vi "数据主动和反控发送.vi"() -> ()   [LabVIEW 2016, in "数据传输系统.lvlib"]
uses:
  <vilib>/ptbypt/NI_PtbyPt.lvlib
panel:
  out "QN":string
  out "队列中元素数量":i32
  out "元素":cluster{"命令编码CN":string, "QN":string}[](array[cluster])
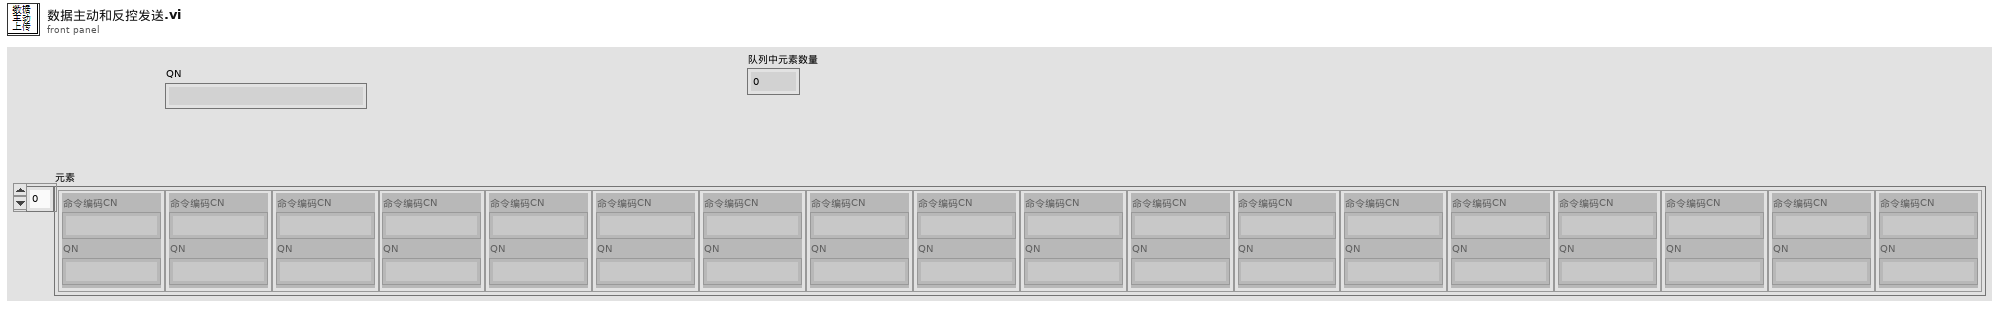
[diagram p1: front panel]
types:
  T1 = enum16{"00点", "01点", "02点", "03点", "04点", "05点", "06点", "07点", "08点", "09点", "10点", "11点", "12点", "13点", "14点", "15点", "16点", "17点", "18点", "19点", "20点", "21点", "22点", "23点"}
  T2 = enum16{"关闭", "星期日", "星期一", "星期二", "星期三", "星期四", "星期五", "星期六"}
  T3 = typedef "LVDateTimeRec.ctl" = cluster{"秒数的小数部分":dbl, "秒":i32, "分":i32, "时":i32, "日":i32, "月":i32, "年":i32, "天数（周）":i32, "天数（年）":i32, "DST":i32}
  T4 = cluster{"[0]":string, "[1]":string, "[2]":string, "[3]":string, "[4]":string, "[5]":string, "[6]":string, "[7]":string, "[8]":string, "[9]":string, "[10]":string, "[11]":string, "[12]":string, "[13]":string, "[14]":string, "[15]":string, "[16]":string, "[17]":string, "[18]":string, "[19]":string, "[20]":string, "[21]":string, "[22]":string, "[23]":string, "[24]":string, "[25]":string, "[26]":string}
  T5 = cluster{"CODMn":bool, "CODCr":bool, "DO":bool, "铜":bool, "PH":bool, "氨氮":bool, "比电导率":bool, "水温":bool, "COD":bool, "浊度":bool, "总氮":bool, "总磷":bool, "叶绿素a":bool, "藻密度":bool, "水位":bool, "流速":bool, "瞬时流量":bool, "累积流量":bool, "亚硝酸盐":bool, "硫化物":bool, "ORP":bool, "铅":bool, "镉":bool, "锌":bool, "镍":bool, "锰":bool, "汞":bool}
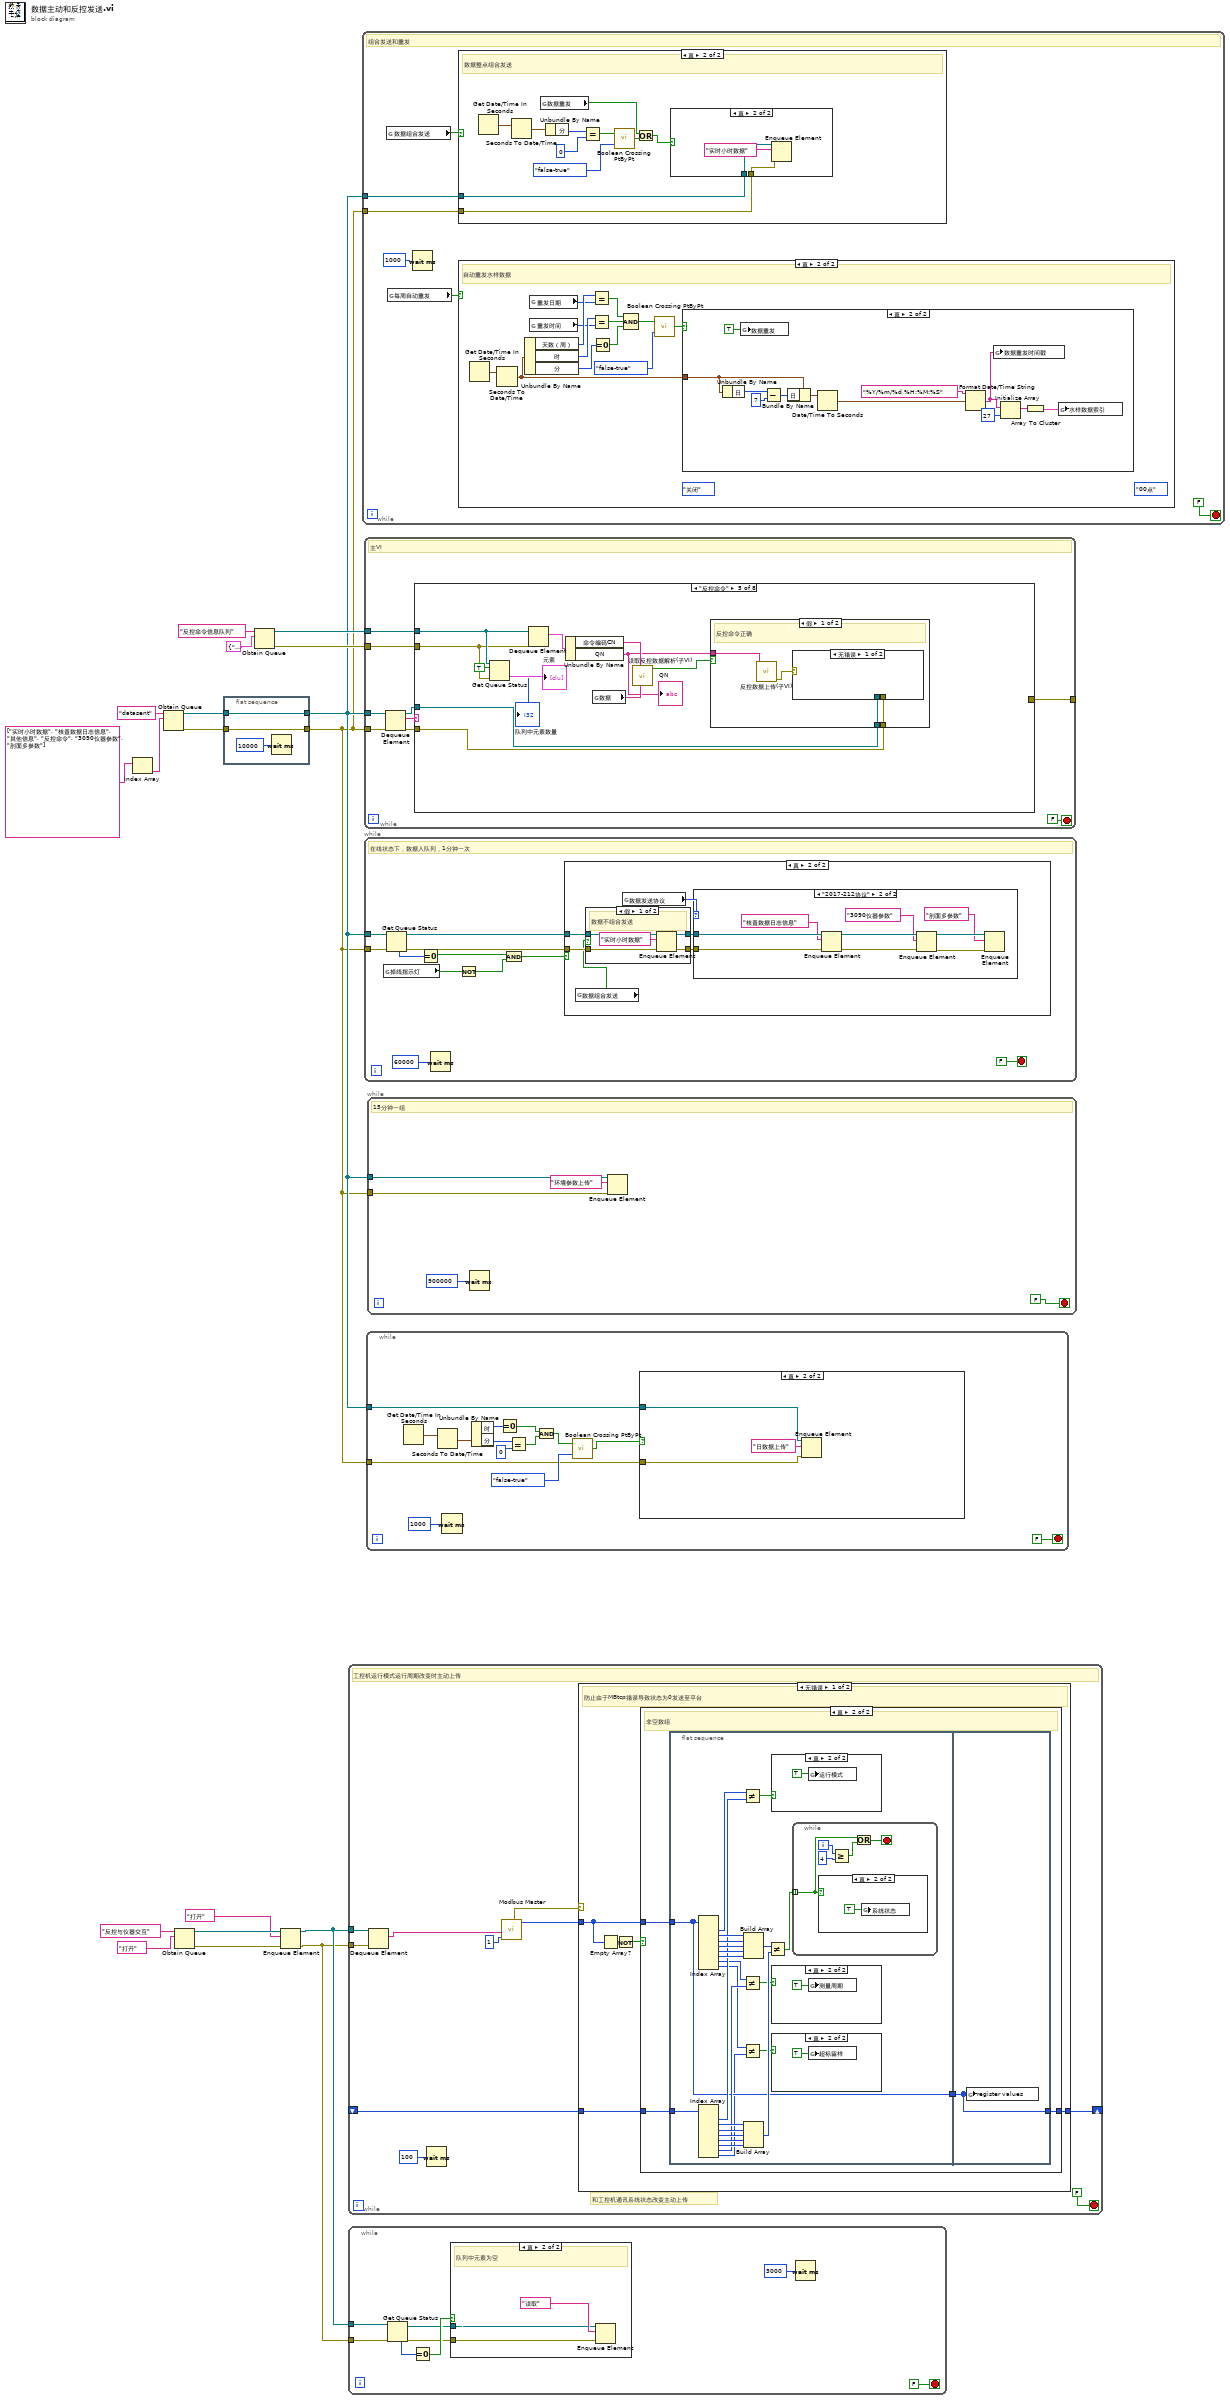
[diagram p0: block diagram]
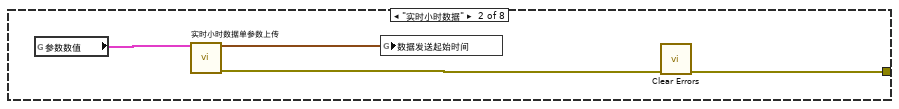
[diagram p18: hidden frame]
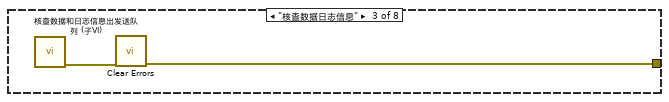
[diagram p19: hidden frame]
diagram:
  n1 = Index Array(array=string[] ["实时小时数据", "核查数据日志信息", "其他信息", "反控命令", "3090仪器参数", "剖面多参数"]) -> (element=w3:string)  [unwired: 1 in]
  n2 = Obtain Queue(name (unnamed)="datasent" ("名称（未命名）"), element data type=w3) -> (queue out=w17:refnum<queue>, error out=w16:errorcluster)  [unwired: 3 in, 1 out]
  n3 = Obtain Queue(name (unnamed)="反控与仪器交互" ("名称（未命名）"), element data type="打开" ("读取写入选择")) -> (queue out=w9:refnum<queue>, error out=w8:errorcluster)  [unwired: 3 in, 1 out]
  n4 = flat-sequence {
    tunnel: w17 -> [w20]
    tunnel: [w20] -> w2
    tunnel: w16 -> [w19]
    tunnel: [w19] -> w1
    frame #0 {
      n5 = Wait (ms)(milliseconds to wait=u32 10000 ("等待时间（毫秒）")) -> ()  [unwired: 1 out]
    }
  }
  n6 = Obtain Queue(name (unnamed)="反控命令信息队列" ("名称（未命名）"), element data type=cluster{"命令编码CN":string, "QN":string} {"命令编码CN"="", "QN"=""}) -> (queue out=w13:refnum<queue>, error out=w12:errorcluster)  [unwired: 3 in, 1 out]
  n7 = Enqueue Element(queue=w9, element="打开" ("读取写入选择"), error in (no error)=w8) -> (queue out=w7:refnum<queue>, error out=w6:errorcluster)  [unwired: 1 in, 1 out]
  n8 = while {
    tunnel: w7 -> [w26]
    tunnel: w6 -> [w25]
    shift-right: [w22] -> _
    shift-left: _ -> [w23]
    stop <- FALSE stop-if-true
    # "和工控机通讯系统状态改变主动上传"
    # "工控机运行模式运行周期改变时主动上传"
    n9 = Dequeue Element(queue=w26, error in (no error)=w25) -> (element=w24:string)  [unwired: 1 in, 3 out]
    n10 = Wait (ms)(milliseconds to wait=u32 100 ("等待时间（毫秒）")) -> ()  [unwired: 1 out]
    n11 = call "Modbus Master.vi"("Unit ID"=u8 1, "读取写入选择"=w24) -> ("register values"=w29:u16[], "error out"=w28:errorcluster)  [unwired: 8 in]
    n12 = case shown="无错误" w28 {
      tunnel: w29 -> [w34 _]
      tunnel: w23 -> [w36 w76]
      tunnel: [w35 w76] -> w22
      frame No Error {
        # "防止由于MBtcp错误导致状态为0发送至平台"
        n13 = Empty Array?(array=w34) -> (empty?=w33:bool)
        n14 = Not(x=w33) -> (.not. x?=w32:bool)
        n15 = case shown="真" w32 {
          tunnel: w36 -> [w37 w40]
          tunnel: [w37 w39] -> w35
          tunnel: w34 -> [_ w38]
          frame False {
          }
          frame True {
            # "非空数组"
            n16 = flat-sequence {
              tunnel: w38 -> [w46]
              tunnel: [w46] -> w41
              tunnel: w40 -> [w42]
              tunnel: w41 -> [w75]
              tunnel: [w75] -> w39
              frame #0 {
                n17 = Index Array(array=w46) -> (element #1=w53:u16, element #2=w65:u16, element #3=w64:u16, element #4=w63:u16, element #5=w62:u16, element #6=w61:u16, element #7=w51:u16, element #8=w45:u16)  [unwired: 8 in]
                n18 = Index Array(array=w42) -> (element #1=w52:u16, element #2=w60:u16, element #3=w59:u16, element #4=w58:u16, element #5=w57:u16, element #6=w56:u16, element #7=w50:u16, element #8=w44:u16)  [unwired: 8 in]
                n19 = Not Equal?(x=w53, y=w52) -> (x != y?=w48:bool)
                n20 = Not Equal?(x=w51, y=w50) -> (x != y?=w49:bool)
                n21 = Not Equal?(x=w45, y=w44) -> (x != y?=w43:bool)
                n22 = Build Array(w65, w64, w63, w62, w61) -> (w55:u16[])
                n23 = Build Array(w60, w59, w58, w57, w56) -> (w54:u16[])
                n24 = Not Equal?(x=w55, y=w54) -> (x != y?=w47:bool[])
                n25 = case shown="真" w48 {
                  frame False {
                  }
                  frame True {
                    n26 = global write "全局1.vi" "运行模式"(TRUE) -> ()
                  }
                }
                n27 = case shown="真" w49 {
                  frame False {
                  }
                  frame True {
                    n28 = global write "全局1.vi" "测量周期"(TRUE ("系统状态改变")) -> ()
                  }
                }
                n29 = case shown="真" w43 {
                  frame False {
                  }
                  frame True {
                    n30 = global write "全局1.vi" "超标留样"(TRUE ("系统状态改变")) -> ()
                  }
                }
                n31 = while {
                  tunnel: w47 -> [w69] mode=indexing
                  i -> [w71]
                  stop <- w67 stop-if-true
                  n32 = case shown="真" w69 {
                    frame False {
                    }
                    frame True {
                      n33 = global write "全局1.vi" "系统状态"(TRUE ("系统状态改变")) -> ()
                    }
                  }
                  n34 = Greater Or Equal?(x=w71, y=4) -> (x >= y?=w68:bool)
                  n35 = Or(x=w69, y=w68) -> (x .or. y?=w67:bool)
                }
              }
              frame #1 {
                n36 = global write "全局1.vi" "register values"(w75) -> ()
              }
            }
          }
        }
      }
      frame Error {
      }
    }
  }
  n37 = while {
    tunnel: w7 -> [w81]
    tunnel: w6 -> [w80]
    stop <- FALSE stop-if-true
    n38 = Get Queue Status(queue=w81, error in (no error)=w80) -> (queue out=w78:refnum<queue>, error out=w77:errorcluster, # elements in queue=w82:i32)  [unwired: 1 in, 5 out]
    n39 = Equal To 0?(x=w82) -> (x = 0?=w79:bool)
    n40 = case shown="真" w79 {
      tunnel: w78 -> [_ w86]
      tunnel: w77 -> [_ w85]
      frame False {
      }
      frame True {
        # "队列中元素为空"
        n41 = Enqueue Element(queue=w86, element="读取" ("读取写入选择"), error in (no error)=w85) -> ()  [unwired: 1 in, 3 out]
      }
    }
    n42 = Wait (ms)(milliseconds to wait=u32 3000 ("等待时间（毫秒）")) -> ()  [unwired: 1 out]
  }
  n43 = while {
    tunnel: w2 -> [w89]
    tunnel: w1 -> [w88]
    stop <- FALSE stop-if-true
    # "组合发送和重发"
    n44 = global read "断电保存全局.vi" "数据组合发送"() -> (w90:bool)
    n45 = global read "断电保存全局.vi" "每周自动重发"() -> (w92:bool)
    n46 = Wait (ms)(milliseconds to wait=u32 1000 ("等待时间（毫秒）")) -> ()  [unwired: 1 out]
    n47 = case shown="真" w92 {
      frame False {
      }
      frame True {
        (unwired) T1."00点"
        (unwired) T2."关闭"
        # "自动重发水样数据"
        n48 = Get Date/Time In Seconds() -> (seconds since 1Jan1904=w120:timestamp)
        n49 = Seconds To Date/Time(time stamp (now)=w120) -> (date time rec=w114:T3)  [unwired: 1 in]
        n50 = Unbundle By Name(w114) -> ("天数（周）"=w119:i32, "时"=w110:i32, "分"=w118:i32)
        n51 = global read "断电保存全局.vi" "重发日期"() -> (w109:T2)
        n52 = global read "断电保存全局.vi" "重发时间"() -> (w108:T1)
        n53 = Equal?(x=w119, y=w109) -> (x = y?=w117:bool)
        n54 = Equal?(x=w110, y=w108) -> (x = y?=w116:bool)
        n55 = Equal To 0?(x=w118) -> (x = 0?=w115:bool)
        n56 = Compound Arithmetic op=AND ("复合运算")(w117, w116, w115) -> (w113:bool)
        n57 = call <vilib>:"Boolean Crossing PtByPt.vi"("direction"=enum16{"either", "false-true", "true-false"}."false-true", "input"=w113) -> ("crossing"=w112:bool)  [unwired: 1 in]
        n58 = case shown="真" w112 {
          tunnel: w114 -> [_ w128]
          frame False {
          }
          frame True {
            n59 = Unbundle By Name(w128) -> ("日"=w131:i32)
            n60 = global write "断电保存全局.vi" "数据重发"(TRUE ("数据重发")) -> ()
            n61 = Subtract(x=w131, y=7) -> (x-y=w129:i32)
            n62 = Bundle By Name(cluster=w128, "日"=w129) -> (w132:T3)
            n63 = Date/Time To Seconds(2:w132) -> (0:w127:timestamp)  [unwired: 1 in]
            n64 = Format Date/Time String(time format string (%c)="%Y/%m/%d %H:%M:%S" ("时间格式字符串(%c)"), seconds (now)=w127) -> (date/time string=w121:string)  [unwired: 1 in]
            n65 = global write "断电保存全局.vi" "数据重发时间戳"(w121) -> ()
            n66 = Initialize Array(w121, 27 ("维数大小")) -> (w123:string[])
            n67 = Array To Cluster(array=w123) -> (cluster=w122:T4)
            n68 = global write "全局 水样时间.vi" "水样数据索引"(w122) -> ()
          }
        }
      }
    }
    n69 = case shown="真" w90 {
      tunnel: w89 -> [_ w95]
      tunnel: w88 -> [_ w94]
      frame False {
      }
      frame True {
        # "数据整点组合发送"
        n70 = Get Date/Time In Seconds() -> (seconds since 1Jan1904=w103:timestamp)
        n71 = Seconds To Date/Time(time stamp (now)=w103) -> (date time rec=w104:T3)  [unwired: 1 in]
        n72 = global read "断电保存全局.vi" "数据重发"() -> (w97:bool)
        n73 = Unbundle By Name(w104) -> ("分"=w102:i32)
        n74 = Equal?(x=w102, y=0) -> (x = y?=w100:bool)
        n75 = call <vilib>:"Boolean Crossing PtByPt.vi"("direction"=enum16{"either", "false-true", "true-false"}."false-true", "input"=w100) -> ("crossing"=w98:bool)  [unwired: 1 in]
        n76 = Or(x=w97, y=w98) -> (x .or. y?=w96:bool)
        n77 = case shown="真" w96 {
          tunnel: w95 -> [_ w106]
          tunnel: w94 -> [_ w105]
          frame False {
          }
          frame True {
            n78 = Enqueue Element(queue=w106, element="实时小时数据" ("元素"), error in (no error)=w105) -> ()  [unwired: 1 in, 3 out]
          }
        }
      }
    }
  }
  n79 = while {
    tunnel: w2 -> [w135]
    tunnel: w1 -> [w134]
    tunnel: w13 -> [w137]
    tunnel: w12 -> [w136]
    tunnel: [w133] -> _
    stop <- FALSE stop-if-true
    # "主VI"
    n80 = Dequeue Element(queue=w135, error in (no error)=w134) -> (queue out=w139:refnum<queue>, element=w140:string, error out=w138:errorcluster)  [unwired: 1 in, 1 out]
    n81 = case shown="\"反控命令\"" w140 {
      tunnel: w139 -> [_ _ _ _ w149 _ _ _]
      tunnel: w138 -> [_ _ _ _ w148 _ _ _]
      tunnel: w137 -> [_ _ _ _ w159 _ _ _]
      tunnel: w136 -> [_ _ _ _ w158 _ _ _]
      tunnel: [_ w142 w146 _ _ w164 w165 w166] -> w133
      frame Default {
      }
      frame "实时小时数据" {
        n82 = global read "全局1.vi" "参数数值"() -> (w144:T5)
        n83 = call "实时小时数据单参数上传.vi"("参数数值"=w144) -> ("数据发送起始时间"=w145:timestamp, "error out"=w143:errorcluster)  [unwired: 13 in]
        n84 = global write "全局1.vi" "数据发送起始时间"(w145) -> ()
        n85 = call <vilib>:"Clear Errors.vi"("error in (no error)"=w143) -> ("error out"=w142:errorcluster)  [unwired: 5 in, 1 out]
      }
      frame "核查数据日志信息" {
        n86 = call "核查数据和日志信息出发送队列 (子VI).vi"() -> ("错误输出"=w147:errorcluster)  [unwired: 11 in]
        n87 = call <vilib>:"Clear Errors.vi"("error in (no error)"=w147) -> ("error out"=w146:errorcluster)  [unwired: 5 in, 1 out]
      }
      frame "其他信息" {
      }
      frame "反控命令" {
        n88 = Get Queue Status(queue=w159, return elements? (F)=TRUE ("返回元素？(F)"), error in (no error)=w158) -> (# elements in queue=→"队列中元素数量":i32, elements=→"元素":cluster{"命令编码CN":string, "QN":string}[])  [unwired: 6 out]
        n89 = Dequeue Element(queue=w159, error in (no error)=w158) -> (element=w155:cluster{"命令编码CN":string, "QN":string})  [unwired: 1 in, 3 out]
        n90 = Unbundle By Name(w155) -> ("命令编码CN"=w154:string, "QN"=w153:string)
        "QN" <- w153
        n91 = global read "全局1.vi" "数据"() -> (w157:string)
        n92 = call "读取反控数据解析(子VI).vi"("数据"=w157, "命令编码CN"=w154) -> ("反控命令错误？"=w156:bool)  [unwired: 7 in, 2 out]
        n93 = case shown="假" w156 {
          tunnel: w153 -> [w163 _]
          tunnel: w149 -> [w161 _]
          tunnel: w148 -> [w160 _]
          frame False {
            # "反控命令正确"
            n94 = call "反控数据上传(子VI).vi"("QN"=w163) -> ("error out"=w162:errorcluster)  [unwired: 10 in]
            n95 = case shown="无错误" w162 {
              tunnel: w161 -> [_ _]
              tunnel: w160 -> [_ _]
              frame No Error {
              }
              frame Error {
              }
            }
          }
          frame True {
            # "反控命令错误"
          }
        }
      }
      frame "3090仪器参数" {
        n96 = call "3090仪器参数上传.vi"() -> ("error out"=w164:errorcluster)  [unwired: 15 in]
      }
      frame "剖面多参数" {
        n97 = call "剖面多参数上传.vi"() -> ("error out"=w165:errorcluster)  [unwired: 15 in]
      }
      frame "环境参数上传" {
        n98 = call "环境参数上传.vi"() -> ("error out"=w166:errorcluster)  [unwired: 15 in]
      }
    }
  }
  n99 = while {
    tunnel: w2 -> [w177]
    tunnel: w1 -> [w176]
    stop <- FALSE stop-if-true
    # "在线状态下，数据入队列，1分钟一次"
    n100 = global read "全局 数据发送重叠.vi" "掉线指示灯"() -> (w170:bool)
    n101 = Get Queue Status(queue=w177, error in (no error)=w176) -> (queue out=w174:refnum<queue>, error out=w173:errorcluster, # elements in queue=w175:i32)  [unwired: 1 in, 5 out]
    n102 = Equal To 0?(x=w175) -> (x = 0?=w168:bool)
    n103 = Wait (ms)(milliseconds to wait=u32 60000 ("等待时间（毫秒）")) -> ()  [unwired: 1 out]
    n104 = Not(x=w170) -> (.not. x?=w167:bool)
    n105 = And(x=w168, y=w167) -> (x .and. y?=w169:bool)
    n106 = case shown="真" w169 {
      tunnel: w174 -> [_ w183]
      tunnel: w173 -> [_ w182]
      frame False {
      }
      frame True {
        n107 = global read "断电保存全局.vi" "数据组合发送"() -> (w178:bool)
        n108 = case shown="假" w178 {
          tunnel: w183 -> [w188 w190]
          tunnel: w182 -> [w187 w189]
          tunnel: [w186 w190] -> w181
          tunnel: [w185 w189] -> w180
          frame False {
            # "数据不组合发送"
            n109 = Enqueue Element(queue=w188, element="实时小时数据" ("元素"), error in (no error)=w187) -> (queue out=w186:refnum<queue>, error out=w185:errorcluster)  [unwired: 1 in, 1 out]
          }
          frame True {
            # "数据组合发送"
          }
        }
        n110 = global read "断电保存全局.vi" "数据发送协议"() -> (w179:enum16{"2005-212协议", "2017-212协议"})
        n111 = case shown="\"2017-212协议\"" w179 {
          tunnel: w181 -> [_ w199]
          tunnel: w180 -> [_ w198]
          frame "2005-212协议", Default {
          }
          frame "2017-212协议" {
            n112 = Enqueue Element(queue=w199, element="核查数据日志信息" ("元素"), error in (no error)=w198) -> (queue out=w196:refnum<queue>, error out=w195:errorcluster)  [unwired: 1 in, 1 out]
            n113 = Enqueue Element(queue=w196, element="3090仪器参数" ("元素"), error in (no error)=w195) -> (queue out=w193:refnum<queue>, error out=w192:errorcluster)  [unwired: 1 in, 1 out]
            n114 = Enqueue Element(queue=w193, element="剖面多参数" ("元素"), error in (no error)=w192) -> ()  [unwired: 1 in, 3 out]
          }
        }
      }
    }
  }
  n115 = while {
    tunnel: w2 -> [w201]
    tunnel: w1 -> [w200]
    stop <- FALSE stop-if-true
    n116 = Get Date/Time In Seconds() -> (seconds since 1Jan1904=w210:timestamp)
    n117 = Seconds To Date/Time(time stamp (now)=w210) -> (date time rec=w211:T3)  [unwired: 1 in]
    n118 = Wait (ms)(milliseconds to wait=u32 1000 ("等待时间（毫秒）")) -> ()  [unwired: 1 out]
    n119 = Unbundle By Name(w211) -> ("时"=w206:i32, "分"=w209:i32)
    n120 = Equal To 0?(x=w206) -> (x = 0?=w205:bool)
    n121 = Equal?(x=w209, y=0) -> (x = y?=w204:bool)
    n122 = And(x=w205, y=w204) -> (x .and. y?=w203:bool)
    n123 = call <vilib>:"Boolean Crossing PtByPt.vi"("direction"=enum16{"either", "false-true", "true-false"}."false-true", "input"=w203) -> ("crossing"=w202:bool)  [unwired: 1 in]
    n124 = case shown="真" w202 {
      tunnel: w201 -> [_ w215]
      tunnel: w200 -> [_ w214]
      frame False {
      }
      frame True {
        n125 = Enqueue Element(queue=w215, element="日数据上传" ("元素"), error in (no error)=w214) -> ()  [unwired: 1 in, 3 out]
      }
    }
  }
  n126 = while {
    tunnel: w2 -> [w218]
    tunnel: w1 -> [w217]
    stop <- FALSE stop-if-true
    # "15分钟一组"
    n127 = Wait (ms)(milliseconds to wait=u32 900000 ("等待时间（毫秒）")) -> ()  [unwired: 1 out]
    n128 = Enqueue Element(queue=w218, element="环境参数上传" ("元素"), error in (no error)=w217) -> ()  [unwired: 1 in, 3 out]
  }
